vi "array gen.vi"(11 "Temperature Control Parameters":T1 {"End Temp" format="%.2f"; "Temp Step" format="%.2f"; "Start Temp" format="%.2f"}) -> (3 "Temp Array":dbl[](array[numeric]), 8 "too low":bool)   [LabVIEW 2017]
uses:
  typedefs/temp control params.ctl
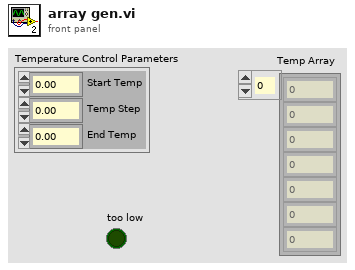
[diagram p1: front panel]
types:
  T1 = typedef "temp control params.ctl" = cluster{"Start Temp":dbl, "Temp Step":dbl, "End Temp":dbl}
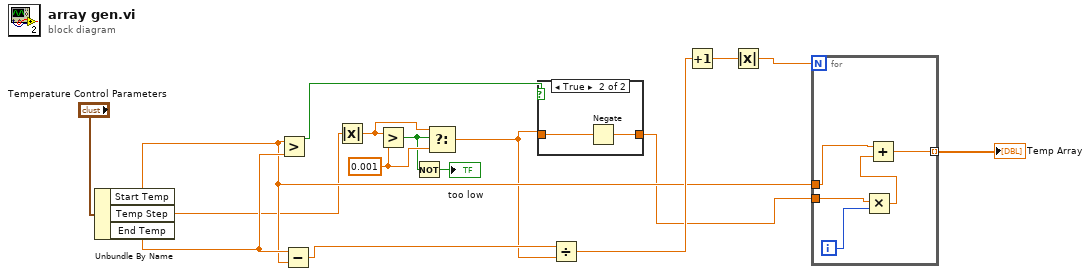
[diagram p0: block diagram]
diagram:
  w7 = 0.001
  n1 = Unbundle By Name("Temperature Control Parameters") -> ("Start Temp"=w10:dbl, "Temp Step"=w8:dbl, "End Temp"=w11:dbl)
  n2 = Greater?(x=w10, y=w11) -> (0:w12:bool)
  n3 = Subtract(x=w11, y=w10) -> (x-y=w15:dbl)
  n4 = Absolute Value(x=w8) -> (abs(x)=w6:dbl)
  n5 = Greater?(x=w6, y=w7) -> (0:w5:bool)
  n6 = Not(x=w5) -> (.not. x?=→"too low":bool)
  n7 = Select(t=w6, s=w5, f=w7) -> (s? t:f=w3:dbl)
  n8 = case shown="True" w12 {
    tunnel: w3 -> [w17 w19]
    tunnel: [w17 w18] -> w9
    frame False {
    }
    frame True {
      n9 = Negate(x=w19) -> (-x=w18:dbl)
    }
  }
  n10 = Divide(x=w15, y=w3) -> (x/y=w14:dbl)
  n11 = Increment(x=w14) -> (x+1=w2:dbl)
  n12 = Absolute Value(x=w2) -> (abs(x)=w1:dbl)
  n13 = for {
    N: w1 -> [_]
    tunnel: w10 -> [w22]
    tunnel: w9 -> [w21]
    tunnel: [w20] -> w13 mode=indexing
    i -> [w24]
    n14 = Multiply(x=w21, y=w24) -> (x*y=w23:dbl)
    n15 = Add(x=w22, y=w23) -> (x+y=w20:dbl)
  }
  "Temp Array" <- w13
